vi "DBBSJWrRecord.vi"(8 "error in":errorcluster caption="错误输入", 10 "String":string) -> (0 "error out":errorcluster caption="错误输出", 1 "SN":string, 2 "ICCID":string, 3 "ReportStr":string, 4 "Result":string[](array[string]))   [LabVIEW 2013]
uses:
  <vilib>/addons/database/Connection.llb/DB Tools Open Connec (String).vi
  <vilib>/addons/database/Connection.llb/Conn Execute.vi
  <vilib>/addons/database/Recordset.llb/Rec Fetch Recordset Data (R).vi
  <vilib>/addons/database/Recordset.llb/Rec Destroy - Connection.vi
  <vilib>/addons/database/NI_Database_API.lvlib
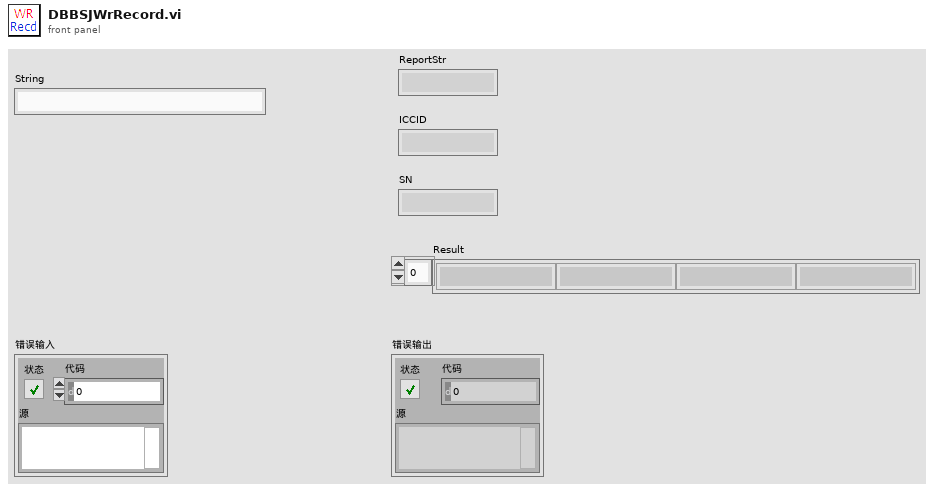
[diagram p1: front panel]
types:
  T1 = typedef "NI_Database_API.lvlib/Conn ObjectReference.ctl" = refnum<k1>
  T2 = typedef "NI_Database_API.lvlib/Rec ObjectReference.ctl" = refnum<k1>
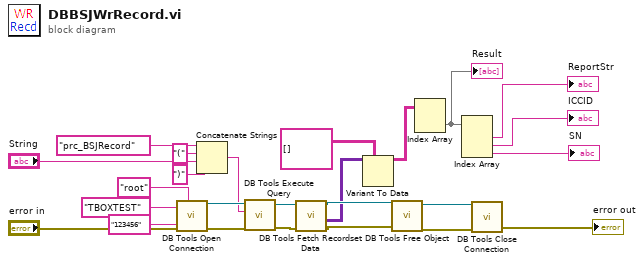
[diagram p0: block diagram]
diagram:
  n1 = call-poly <vilib>:"DB Tools Open Connection.vi"("password"="123456", "userID"="root", "error in (no error)"="error in", "connection information"="TBOXTEST" ("元素")) -> ("error out"=w22:errorcluster, "connection reference"=w23:T1)  [unwired: 4 in]
  n2 = Concatenate Strings("prc_BSJRecord" ("SQL query"), "(" ("字符串"), "String", ")" ("字符串")) -> (w15:string)
  n3 = call-poly <vilib>:"DB Tools Execute Query.vi"("error in (no error)"=w22, "SQL query"=w15, "connection reference"=w23) -> ("error out"=w11:errorcluster, "recordset reference"=w12:T2)  [unwired: 5 in]
  n4 = call-poly <vilib>:"DB Tools Fetch Recordset Data.vi"("error in (no error)"=w11, "recordset reference"=w12) -> ("error out"=w10:errorcluster, "recordset data"=w8:variant[][], "recordset reference out"=w9:T2)  [unwired: 3 in]
  n5 = Variant To Data(type=string[][] [] ("数组"), Variant=w8) -> (data=w7:string[][])  [unwired: 1 in, 1 out]
  n6 = call-poly <vilib>:"DB Tools Free Object.vi"("error in (no error)"=w10, "recordset reference"=w9) -> ("error out"=w21:errorcluster, "connection reference"=w20:T1)  [unwired: 8 in]
  n7 = Index Array(array=w7) -> (element=w4:string[])  [unwired: 2 in]
  "Result" <- w4
  n8 = Index Array(array=w4) -> (element #1=→"ReportStr":string, element #2=→"ICCID":string, element #3=→"SN":string)  [unwired: 3 in]
  n9 = call <vilib>:"DB Tools Close Connection.vi"("error in (no error)"=w21, "connection reference"=w20) -> ("error out"=→"error out":errorcluster)  [unwired: 5 in]
